vi "Increment Read Index.vi"(0 "TDMS In":refnum<k34>, 5 "Increment(1)":u64=1, 11 "Error In":errorcluster) -> (4 "TDMS Out":refnum<k34>, 6 "Read Index":i64, 15 "Error Out":errorcluster)   [LabVIEW 2015, in "Teaching File.lvlib"]
doc: "Increment the value of the <b>Read_Index</b> sample pointer. This pointer is used as the index of the most recent sample to be read. If 0 is wired as the increment, this VI can be used to read the current <b>Read_Index</b> value."
uses:
  Teaching File.lvlib
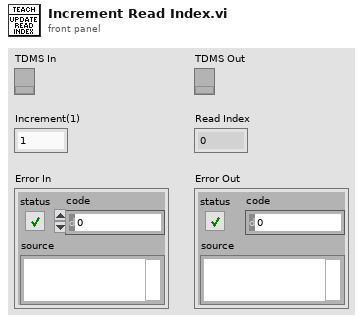
[diagram p1: front panel]
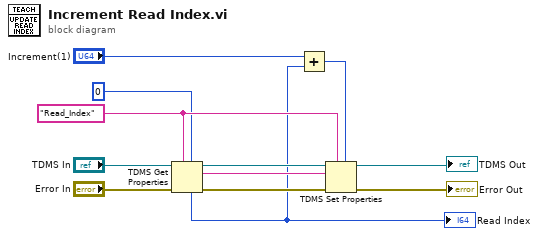
[diagram p0: block diagram]
diagram:
  w10 = "Read_Index" ("property name")
  n1 = TDMS Get Properties(5:i64 0, 7:w10, 8:"Error In", 11:"TDMS In") -> (0:w7:errorcluster, 2:w8:string, 3:w9:refnum<k34>, 4:w3:i64)  [unwired: 2 in, 2 out]
  "Read Index" <- w3
  n2 = Add(x="Increment(1)", y=w3) -> (x+y=w2:u64)
  n3 = TDMS Set Properties(5:w2, 7:w10, 8:w7, 10:w8, 11:w9) -> (0:→"Error Out":errorcluster, 3:→"TDMS Out":refnum<k34>)  [unwired: 1 in, 2 out]
